vi "niRFUtil WFM Linear Feedback Shift Register.vi"(1 "LFSR Polynomial":T1 min=0, 3 "Bit Stream In":T1 min=0, 4 "Initial LFSR Value":T1 min=0) -> (5 "Final LFSR Value":T1 min=0, 6 "Bit Stream Out":T1 min=0)   [LabVIEW 2015, in "niRFUtil.lvlib"]
uses:
  niRFUtil.lvlib
  Includes/niRFUtil INC Bit Array.ctl
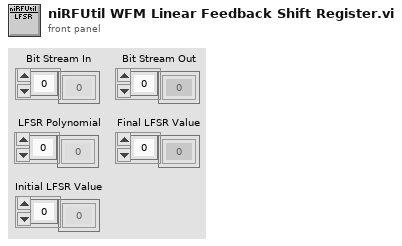
[diagram p1: front panel]
types:
  T1 = typedef "niRFUtil.lvlib/niRFUtil INC Bit Array.ctl" = i8[]
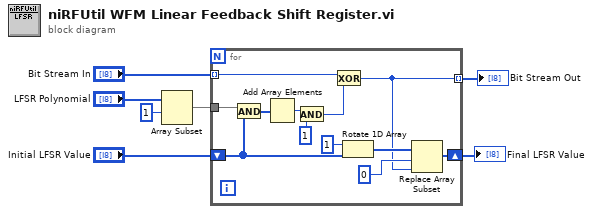
[diagram p0: block diagram]
diagram:
  n1 = Array Subset(array="LFSR Polynomial", index=i8 1) -> (w3:T1)  [unwired: 1 in]
  n2 = for {
    tunnel: "Bit Stream In" -> [w15] mode=indexing
    shift-right: [w9] -> w4
    shift-left: "Initial LFSR Value" -> [w10]
    tunnel: w3 -> [w19]
    tunnel: [w8] -> w1 mode=indexing
    n3 = And(x=w19, y=w10) -> (x .and. y?=w18:i8[])
    n4 = Add Array Elements(numeric array=w18) -> (sum=w17:i8)
    n5 = And(x=w17, y=i8 1) -> (x .and. y?=w14:i8)
    n6 = Exclusive Or(1:w14, 2:w15) -> (0:w8:i8)
    n7 = Rotate 1D Array(1:w10, 2:1 ("n")) -> (0:w12:T1)
    n8 = Replace Array Subset(array=w12, new element=w8, index=0) -> (w9:T1)
  }
  "Bit Stream Out" <- w1
  "Final LFSR Value" <- w4
